vi "P1E1 ZAL 2015640414.vi"() -> ()   [LabVIEW 2016]
panel:
  out "XNOR":bool
  out "XOR":bool
  out "NOR":bool
  out "OR":bool
  out "NAND":bool
  out "AND":bool
  in  "X2":bool
  in  "X1":bool
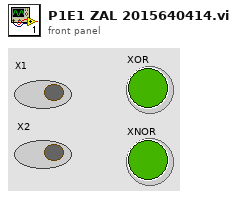
[diagram p1: front panel]
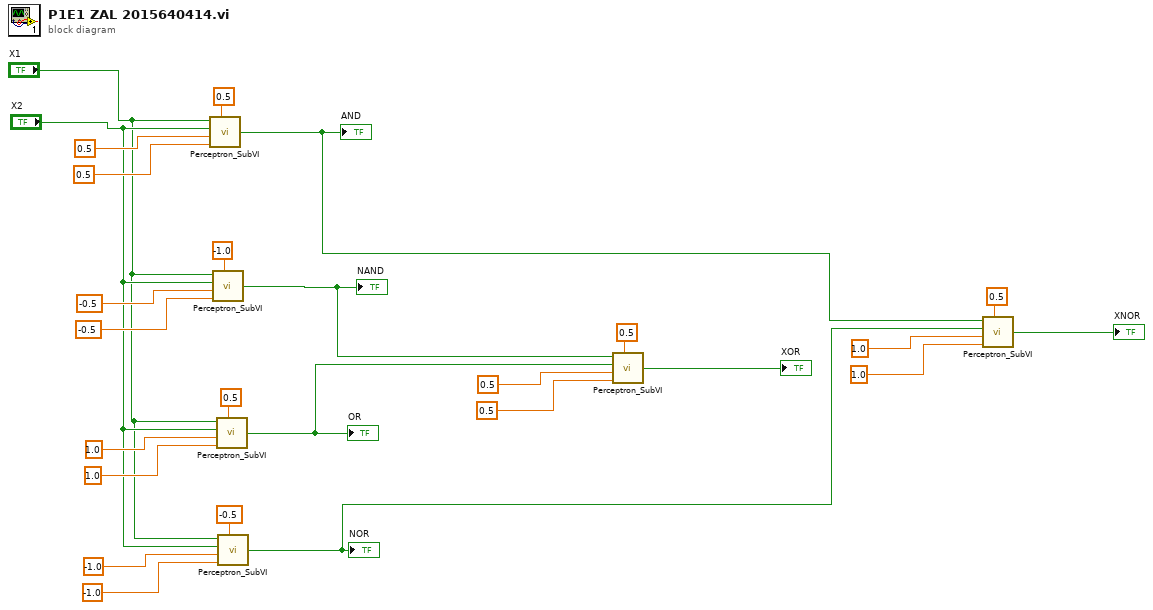
[diagram p0: block diagram]
diagram:
  n1 = call "Perceptron_SubVI.vi"("X1"="X1", "X2"="X2", "W1"=0.5, "W2"=0.5, "Theta"=0.5) -> ("A"=w2:bool)
  "AND" <- w2
  n2 = call "Perceptron_SubVI.vi"("X1"="X1", "X2"="X2", "W1"=-0.5, "W2"=-0.5, "Theta"=-1.0) -> ("A"=w7:bool)
  "NAND" <- w7
  n3 = call "Perceptron_SubVI.vi"("X1"="X1", "X2"="X2", "W1"=1.0, "W2"=1.0, "Theta"=0.5) -> ("A"=w8:bool)
  "OR" <- w8
  n4 = call "Perceptron_SubVI.vi"("X1"="X1", "X2"="X2", "W1"=-1.0, "W2"=-1.0, "Theta"=-0.5) -> ("A"=w3:bool)
  "NOR" <- w3
  n5 = call "Perceptron_SubVI.vi"("X1"=w7, "X2"=w8, "W1"=0.5, "W2"=0.5, "Theta"=0.5) -> ("A"=→"XOR":bool)
  n6 = call "Perceptron_SubVI.vi"("X1"=w2, "X2"=w3, "W1"=1.0, "W2"=1.0, "Theta"=0.5) -> ("A"=→"XNOR":bool)
